vi "CRC.vi"(9 "length":i32=496, 10 "index":i32=20, 11 "DS5CalibrationCoefficientsTable":u8[](array[numeric])=[21, 0, 0, 0, 3, 0, 25, 0, 240, 1, 0, 0, 0, 4, 0, 4, 169, 238, 63, 236, 156, 141, 55, 63, 113, 190, 162, 63, 135, 142, 252, 62, 9, 233, 5, 63, 31, 150, 10, 62, 55, 118, 207, 190, 113, 68, 102, 58, 249, 138, 146, 186, 37, 191, 183, 62, 140, 183, 56, 63, 9, 210, 163, 63, 166, 65, 2, 63, 224, 139, 1, 63, 100, 118, 2, 62, 234, 150, 203, 190, 17, 251, 198, 57, 162, 214, 21, 187, 174, 168, 180, 62, 233, 255, 127, 63, 123, 123, 122, 58, 169, 40, 178, 186, 91, 254, 122, 186, 231, 255, 127, 63, 249, 16, 188, 186, 151, 250, 177, 58, 148, 60, 188, 58, 223, 255, 127, 63, 253, 254, 127, 63, 187, 169, 2, 187, 133, 7, 170, 187, 170, 38, 3, 59, 205, 255, 127, 63, 195, 120, 187, 58, 120, 239, 169, 59, 115, 212, 188, 186, 13, 255, 127, 63, 197, 83, 91, 194, 1, 0, 0, 0, 0, 0, 0, 0, 0, 0, 0, 0, 0, 0, 0, 0, 0, 0, 0, 0, 0, 0, 0, 0, 0, 0, 0, 0, 0, 0, 0, 0, 0, 0, 0, 0, 0, 0, 0, 0, 0, 0, 0, 0, 0, 0, 0, 0, 0, 0, 0, 0, 0, 0, 0, 0, 0, 0, 0, 0, 0, 0, 0, 0, 0, 0, 0, 0, 0, 0, 0, 0, 0, 0, 0, 0, 0, 0, 0, 0, 0, 0, 0, 0, 0, 0, 0, 0, 0, 0, 0, 0, 27, 157, 178, 68, 27, 157, 178, 68, 254, 246, 109, 68, 45, 3, 11, 68, 207, 38, 110, 68, 207, 38, 110, 68, 169, 164, 30, 68, 145, 89, 185, 67, 138, 196, 30, 68, 138, 196, 30, 68, 225, 48, 158, 67, 23, 34, 119, 67, 138, 196, 30, 68, 138, 196, 30, 68, 225, 48, 210, 67, 23, 34, 119, 67, 207, 38, 238, 67, 207, 38, 238, 67, 169, 164, 158, 67, 145, 89, 57, 67, 138, 196, 158, 67, 138, 196, 158, 67, 225, 48, 82, 67, 23, 34, 247, 66, 138, 196, 158, 67, 138, 196, 158, 67, 225, 48, 30, 67, 23, 34, 247, 66, 27, 157, 178, 67, 27, 157, 178, 67, 254, 246, 109, 67, 45, 3, 11, 67, 115, 78, 132, 68, 115, 78, 132, 68, 17, 126, 30, 68, 190, 241, 205, 67, 27, 157, 50, 68, 27, 157, 50, 68, 254, 246, 237, 67, 45, 3, 139, 67, 0, 0, 0, 0, 0, 0, 0, 0, 0, 0, 0, 0, 0, 0, 0, 0, 0, 0, 0, 0, 0, 0, 0, 0, 0, 0, 0, 0, 0, 0, 0, 0, 0, 0, 0, 0, 0, 0, 0, 0, 0, 0, 0, 0, 0, 0, 0, 0, 0, 0, 0, 0, 0, 0, 0, 0, 0, 0, 0, 0, 0, 0, 0, 0, 0, 0, 0, 0, 0, 0, 0, 0, 0, 0, 0, 0, 0, 0, 0, 0, 0, 0, 0, 0, 0, 0, 0, 0, 0, 0, 0, 0, 0, 0, 0, 0, 0, 0, 0, 0, 105, 207, 27, 52, 0, 14, 0, 128, 67, 0, 58, 0, 92, 0, 80, 0, 114, 0, 111, 0, 103, 0, 114, 0, 97, 0, 109, 0, 32, 0, 70, 0, 105, 0, 108, 0, 101, 0, 115, 0, 92, 0, 78, 0, 97, 0, 116, 0, 105, 0, 111, 0, 110, 0, 97, 0, 108, 0, 32, 0, 73, 0, 110, 0, 115, 0, 116, 0, 114, 0, 117, 0, 109, 0, 101, 0, 110, 0, 116, 0, 115, 0, 92, 0, 76, 0, 97, 0, 98, 0, 86, 0, 73, 0, 69, 0, 87, 0, 32, 0, 50, 0, 48, 0, 49, 0, 54, 0, 92, 0, 76, 0, 97, 0, 98, 0, 86, 0, 73, 0, 69, 0, 87, 0, 46, 0, 101, 0, 120, 0, 101, 0, 0, 0, 114, 0, 101, 0, 92, 0, 112, 0, 110, 0, 103, 0, 46, 0, 108, 0, 108, 0, 98, 0, 0, 0, 0, 0, 0, 0, 0, 0, 0, 0, 0, 0, 0, 0, 0, 0, 0, 0, 0, 0, 0, 0, 0, 0, 0, 0, 0, 0, 0, 0, 0, 0, 0, 0, 0, 0, 0, 0, 0, 0, 0, 0, 0, 0, 0, 0, 0, 0, 0, 0, 0, 0, 0, 0, 0, 0, 0, 0, 0, 0, 0, 0, 0, 0, 0, 0, 0, 0, 0, 0, 0, 0, 0, 0, 0, 0, 0, 0, 0, 0, 0, 0, 0, 0, 0, 0, 0, 0, 0, 0, 0, 0, 0, 0, 0, 0, 0, 0, 0, 0, 0, 0, 0, 0, 0, 0, 0, 0, 0, 0, 0, 0, 0, 0, 0, 0, 0, 0, 0, 0, 0, 0, 0, 0, 0, 0, 0, 0, 0, 0, 0, 0, 0, 0, 0, 0, 0, 0, 0, 0, 0, 0, 0, 0, 0, 0, 0, 0, 0, 0, 0, 0, 0, 0, 0, 0, 0, 0, 0, 0, 0, 0, 0, 0, 0, 0, 0, 0, 0, 0, 0, 0, 0, 0, 0, 0, 0, 0, 0, 0, 0, 0, 0, 0, 0, 0, 0, 0, 0, 0, 0, 0, 0, 0, 0, 0, 0, 0, 0, 0, 0, 0, 0, 0, 0, 0, 0, 0, 0, 0, 0, 0, 0, 0, 0, 0, 0, 0, 0, 0, 0, 0, 0, 0, 0, 0, 0, 0, 0, 0, 0, 0, 0, 0, 0, 0, 0, 0, 0, 0, 0, 0, 0, 0, 0, 0, 0, 0, 0, 0, 0, 0, 0, 0, 0, 0, 0, 0, 0, 0, 0, 0, 0, 0, 0, 0, 0, 0, 0, 0, 0, 0, 0, 0, 0, 0, 0, 0, 0, 0, 0, 0, 0, 0, 0, 0, 0, 0, 0, 0, 0, 0, 0, 0, 0, 0, 0, 0, 0, 0, 0, 0, 0, 0, 0, 0, 0, 0, 0, 0, 0, 0, 0, 0, 0, 0, 0, 0, 0, 0, 0, 0, 0, 0, 0, 0, 0, 0, 0, 0, 0, 0, 0, 0, 0, 0, 0, 0, 0, 0, 0, 0, 0, 0, 0, 0, 0, 0, 0, 0] format="%x") -> (2 "CRC array":u8[](array[numeric]), 3 "CRC output":u32=3963612841 format="%x")   [LabVIEW 2017, in "libRealSense3.lvlib"]
uses:
  libRealSense3.lvlib
panel:
  out "Calibration table":T1={"version"=3, "table type"=60479, "table size"=496, "full version"=67109888, "crc32"=3963612841, "baseline"=-54.831806, "model"=1, "fx left"=917.7658, "fy left"=915.4345, "px left"=631.39185, "py left"=376.6227, "py right"=364.3492, "px right"=651.2822, "fy right"=921.49005, "fx right"=923.5849, "k left"=[0.13533829, -0.40519878, 0.0008784002, -0.0011180333, 0.3588802], "k right"=[0.12740475, -0.39763576, 0.00037952562, -0.0022863527, 0.35284942], "RLeft"=[0.9999986, 0.0009555143, -0.001359244, -0.0009574645, 0.9999985, -0.001434832, 0.001357871, 0.0014361315, 0.99999803], "Rright"=[0.99998456, -0.0019937593, -0.0051888847, 0.002001206, 0.99999696, 0.0014302958, 0.0051860176, -0.0014406577, 0.9999855], "uint8 reserved1"=[0, 0, 0, 0, 0, 0, 0, 0, 0, 0, 0, 0, 0, 0, 0, 0, 0, 0, 0, 0, 0, 0, 0, 0, 0, 0, 0, 0, 0, 0, 0, 0, 0, 0, 0, 0, 0, 0, 0, 0, 0, 0, 0, 0, 0, 0, 0, 0, 0, 0, 0, 0, 0, 0, 0, 0, 0, 0, 0, 0, 0, 0, 0, 0, 0, 0, 0, 0, 0, 0, 0, 0, 0, 0, 0, 0, 0, 0, 0, 0, 0, 0, 0, 0, 0, 0, 0, 0], "uint8 reserved2"=[0, 0, 0, 0, 0, 0, 0, 0, 0, 0, 0, 0, 0, 0, 0, 0, 0, 0, 0, 0, 0, 0, 0, 0, 0, 0, 0, 0, 0, 0, 0, 0, 0, 0, 0, 0, 0, 0, 0, 0, 0, 0, 0, 0, 0, 0, 0, 0, 0, 0, 0, 0, 0, 0, 0, 0, 0, 0, 0, 0, 0, 0, 0, 0], "1920x1080"=[1428.9095, 1428.9095, 951.85925, 556.0496], "1280x720"=[952.6064, 952.6064, 634.5728, 370.69974], "640x480"=[635.0709, 635.0709, 316.38187, 247.13316], "848x480"=[635.0709, 635.0709, 420.38187, 247.13316], "640x360"=[476.3032, 476.3032, 317.2864, 185.34987], "424x240"=[317.53546, 317.53546, 210.19093, 123.56658], "320x240"=[317.53546, 317.53546, 158.19093, 123.56658], "480x270"=[357.2274, 357.2274, 237.96481, 139.0124], "1280x800"=[1058.4515, 1058.4515, 633.9698, 411.8886], "960x540"=[714.4548, 714.4548, 475.92963, 278.0248], "Reserved1"=[714.4548, 714.4548, 475.92963, 278.0248], "Reserved 2"=[714.4548, 714.4548, 475.92963, 278.0248]} {"crc32" format="%x"}
  out "iteration":i32=495
  out "CRC Array":u32[](array[numeric])=[0, 1996959894, 3993919788, 2567524794, 124634137, 1886057615, 3915621685, 2657392035, 249268274, 2044508324, 3772115230, 2547177864, 162941995, 2125561021, 3887607047, 2428444049, 498536548, 1789927666, 4089016648, 2227061214, 450548861, 1843258603, 4107580753, 2211677639, 325883990, 1684777152, 4251122042, 2321926636, 335633487, 1661365465, 4195302755, 2366115317, 997073096, 1281953886, 3579855332, 2724688242, 1006888145, 1258607687, 3524101629, 2768942443, 901097722, 1119000684, 3686517206, 2898065728, 853044451, 1172266101, 3705015759, 2882616665, 651767980, 1373503546, 3369554304, 3218104598, 565507253, 1454621731, 3485111705, 3099436303, 671266974, 1594198024, 3322730930, 2970347812, 795835527, 1483230225, 3244367275, 3060149565, 1994146192, 31158534, 2563907772, 4023717930, 1907459465, 112637215, 2680153253, 3904427059, 2013776290, 251722036, 2517215374, 3775830040, 2137656763, 141376813, 2439277719, 3865271297, 1802195444, 476864866, 2238001368, 4066508878, 1812370925, 453092731, 2181625025, 4111451223, 1706088902, 314042704, 2344532202, 4240017532, 1658658271, 366619977, 2362670323, 4224994405, 1303535960, 984961486, 2747007092, 3569037538, 1256170817, 1037604311, 2765210733, 3554079995, 1131014506, 879679996, 2909243462, 3663771856, 1141124467, 855842277, 2852801631, 3708648649, 1342533948, 654459306, 3188396048, 3373015174, 1466479909, 544179635, 3110523913, 3462522015, 1591671054, 702138776, 2966460450, 3352799412, 1504918807, 783551873, 3082640443, 3233442989, 3988292384, 2596254646, 62317068, 1957810842, 3939845945, 2647816111, 81470997, 1943803523, 3814918930, 2489596804, 225274430, 2053790376, 3826175755, 2466906013, 167816743, 2097651377, 4027552580, 2265490386, 503444072, 1762050814, 4150417245, 2154129355, 426522225, 1852507879, 4275313526, 2312317920, 282753626, 1742555852, 4189708143, 2394877945, 397917763, 1622183637, 3604390888, 2714866558, 953729732, 1340076626, 3518719985, 2797360999, 1068828381, 1219638859, 3624741850, 2936675148, 906185462, 1090812512, 3747672003, 2825379669, 829329135, 1181335161, 3412177804, 3160834842, 628085408, 1382605366, 3423369109, 3138078467, 570562233, 1426400815, 3317316542, 2998733608, 733239954, 1555261956, 3268935591, 3050360625, 752459403, 1541320221, 2607071920, 3965973030, 1969922972, 40735498, 2617837225, 3943577151, 1913087877, 83908371, 2512341634, 3803740692, 2075208622, 213261112, 2463272603, 3855990285, 2094854071, 198958881, 2262029012, 4057260610, 1759359992, 534414190, 2176718541, 4139329115, 1873836001, 414664567, 2282248934, 4279200368, 1711684554, 285281116, 2405801727, 4167216745, 1634467795, 376229701, 2685067896, 3608007406, 1308918612, 956543938, 2808555105, 3495958263, 1231636301, 1047427035, 2932959818, 3654703836, 1088359270, 936918000, 2847714899, 3736837829, 1202900863, 817233897, 3183342108, 3401237130, 1404277552, 615818150, 3134207493, 3453421203, 1423857449, 601450431, 3009837614, 3294710456, 1567103746, 711928724, 3020668471, 3272380065, 1510334235, 755167117] format="%x"
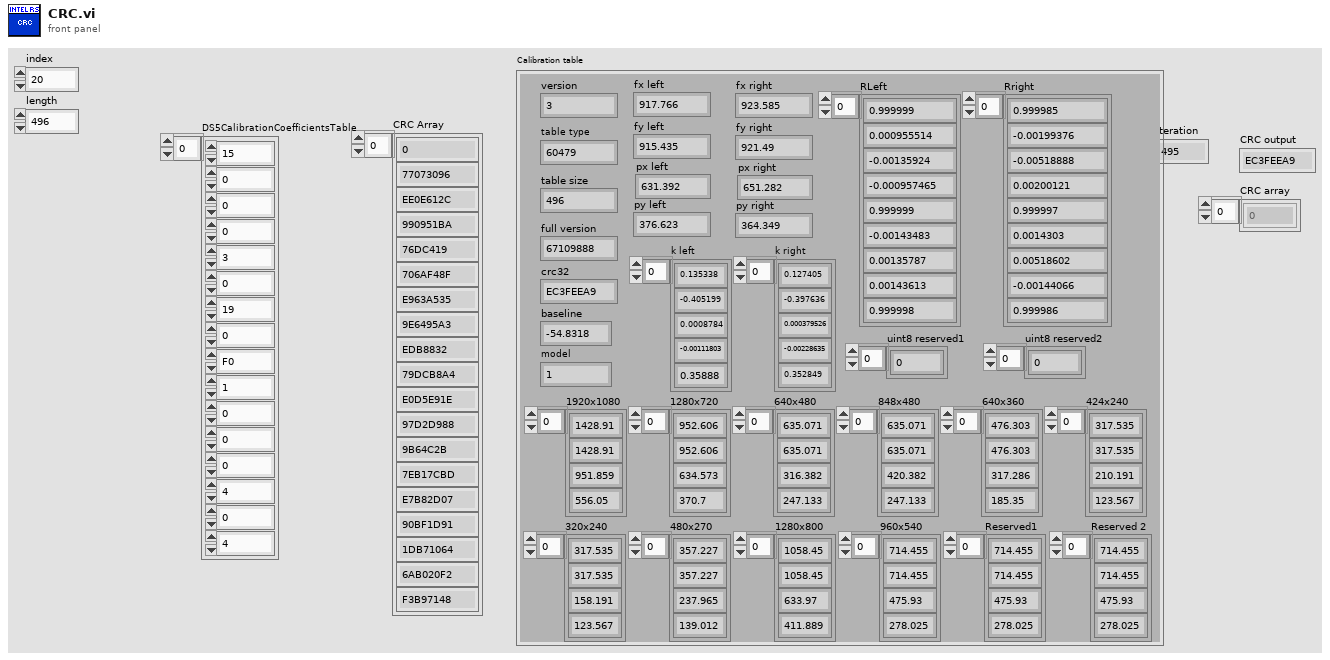
[diagram p1: front panel]
types:
  T1 = cluster{"version":u16, "table type":u16, "table size":u32, "full version":u32, "crc32":u32, "baseline":sgl, "model":u32, "fx left":sgl, "fy left":sgl, "px left":sgl, "py left":sgl, "py right":sgl, "px right":sgl, "fy right":sgl, "fx right":sgl, "k left":sgl[], "k right":sgl[], "RLeft":sgl[], "Rright":sgl[], "uint8 reserved1":u8[], "uint8 reserved2":u8[], "1920x1080":sgl[], "1280x720":sgl[], "640x480":sgl[], "848x480":sgl[], "640x360":sgl[], "424x240":sgl[], "320x240":sgl[], "480x270":sgl[], "1280x800":sgl[], "960x540":sgl[], "Reserved1":sgl[], "Reserved 2":sgl[]}
  T2 = enum16{"big-endian, network order", "native, host order", "little-endian"}
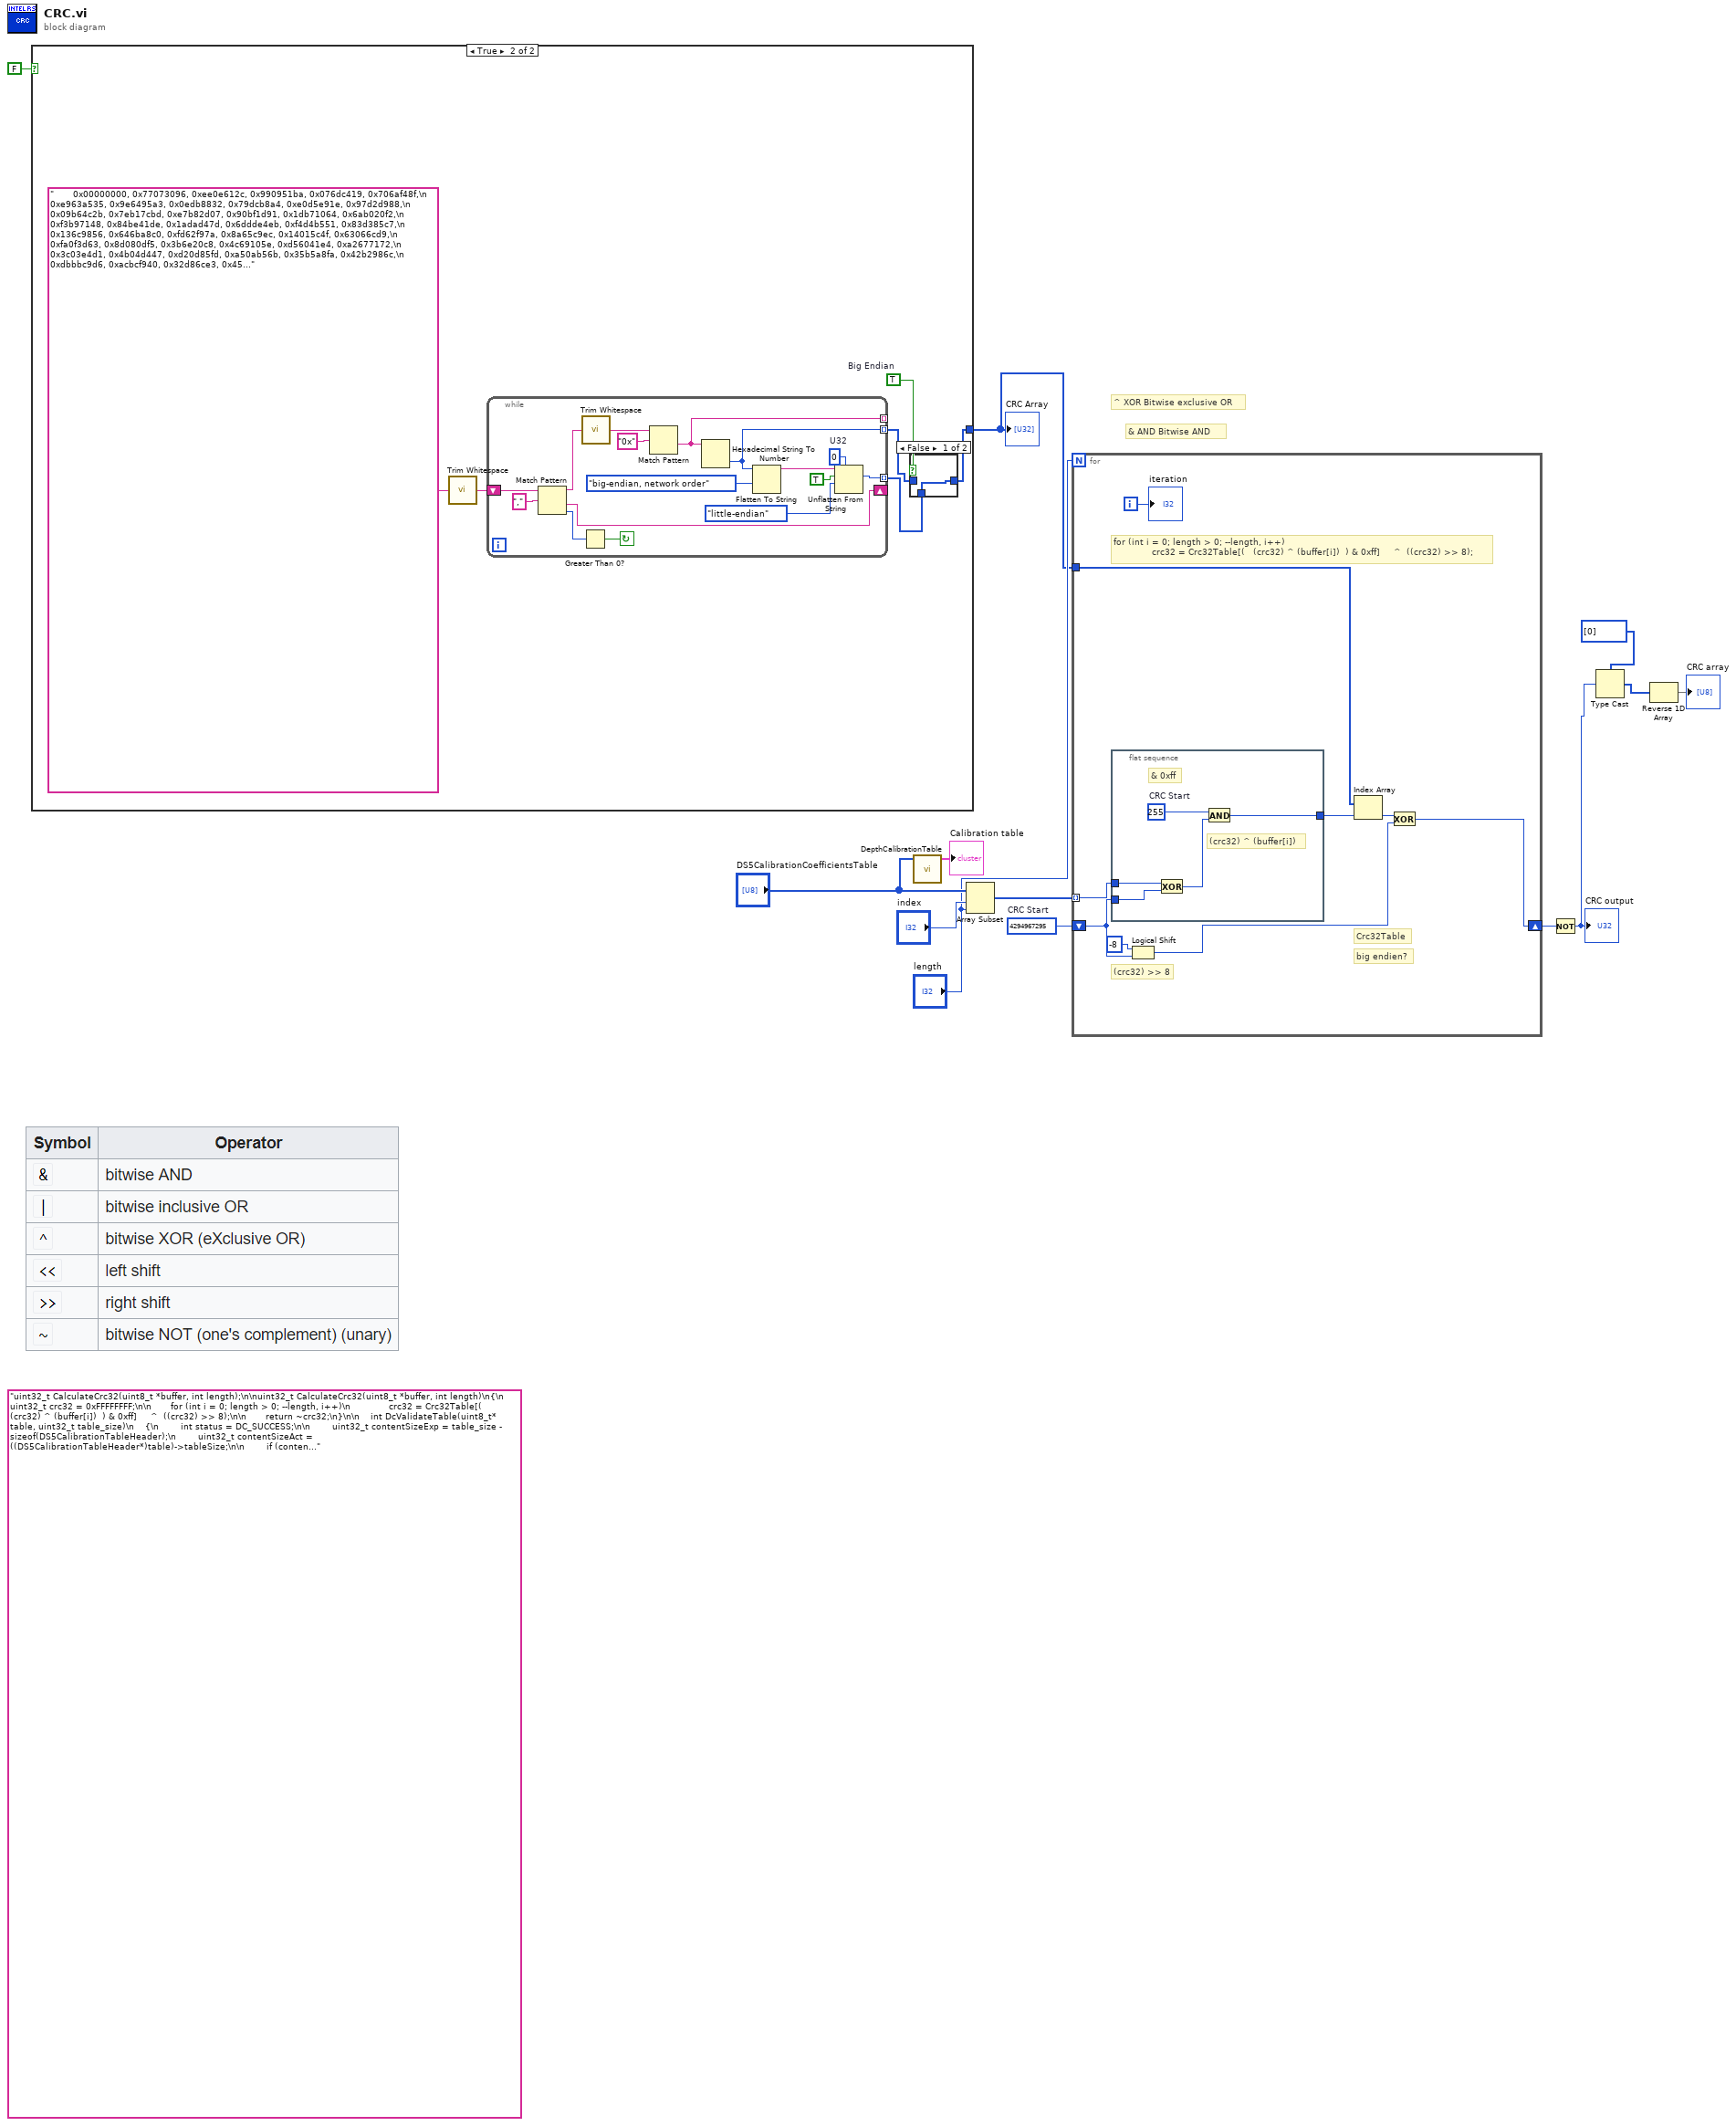
[diagram p0: block diagram]
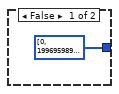
[diagram p2: hidden frame]
diagram:
  w13 = u32 4294967295  # CRC Start
  (unwired) "uint32_t CalculateCrc32(uint8_t *buffer, int length);\n\nuint32_t CalculateCrc32(uint8_t *buffer, int length)\n{\n       uint32_t crc32 = 0xFFFFFFFF;\n\n       for (int i = 0; length > 0; --length, i++)\n              crc32 = Crc32Table[(   (crc32) ^ (buffer[i])  ) & 0xff]     ^  ((crc32) >> 8);\n\n       return ~crc32;\n}\n\n    int DcValidateTable(uint8_t* table, uint32_t table_size)\n    {\n        int status = DC_SUCCESS;\n\n        uint32_t contentSizeExp = table_size - sizeof(DS5CalibrationTableHeader);\n        uint32_t contentSizeAct = ((DS5CalibrationTableHeader*)table)->tableSize;\n\n        if (contentSizeAct > contentSizeExp )\n        {\n            return DC_ERROR_MISMATCH_CAL_TABLE_SIZE;\n        }\n\n        uint8_t* content = table + sizeof(DS5CalibrationTableHeader);\n        uint32_t crc32_comp = CalculateCrc32(content, contentSizeAct);\n        uint32_t crc32_act  = ((DS5CalibrationTableHeader *)table)->crc32;\n\n        if (crc32_act != crc32_comp)\n       {\n            status = DC_ERROR_MISMATCH_CAL_TABLE_CRC;\n        }\n\n        return status;\n       }\n\n\nstruct MMTableHeader\n{\n       uint16_t version;                       //!< Table version\n       uint16_t tableType;                     //!< Table type\n       uint32_t tableSize;                     //!< Table size\n       uint32_t resrved;                       //!< reserved field\n       uint32_t crc32;                         //!< CRC32 of the content\n};\n\n\n\n\n\n\n            status = DcValidateTable(buffer, sizeof(DS5CoefficientsParamsTable));\n"
  # "&\tAND\tBitwise AND"
  # "^\tXOR\tBitwise exclusive OR"
  n1 = case shown="True" FALSE {
    tunnel: [u32[] [0, 1996959894, 3993919788, 2567524794, 124634137, 1886057615, 3915621685, 2657392035, 249268274, 2044508324, 3772115230, 2547177864, 162941995, 2125561021, 3887607047, 2428444049, 498536548, 1789927666, 4089016648, 2227061214, 450548861, 1843258603, 4107580753, 2211677639, 325883990, 1684777152, 4251122042, 2321926636, 335633487, 1661365465, 4195302755, 2366115317, 997073096, 1281953886, 3579855332, 2724688242, 1006888145, 1258607687, 3524101629, 2768942443, 901097722, 1119000684, 3686517206, 2898065728, 853044451, 1172266101, 3705015759, 2882616665, 651767980, 1373503546, 3369554304, 3218104598, 565507253, 1454621731, 3485111705, 3099436303, 671266974, 1594198024, 3322730930, 2970347812, 795835527, 1483230225, 3244367275, 3060149565, 1994146192, 31158534, 2563907772, 4023717930, 1907459465, 112637215, 2680153253, 3904427059, 2013776290, 251722036, 2517215374, 3775830040, 2137656763, 141376813, 2439277719, 3865271297, 1802195444, 476864866, 2238001368, 4066508878, 1812370925, 453092731, 2181625025, 4111451223, 1706088902, 314042704, 2344532202, 4240017532, 1658658271, 366619977, 2362670323, 4224994405, 1303535960, 984961486, 2747007092, 3569037538, 1256170817, 1037604311, 2765210733, 3554079995, 1131014506, 879679996, 2909243462, 3663771856, 1141124467, 855842277, 2852801631, 3708648649, 1342533948, 654459306, 3188396048, 3373015174, 1466479909, 544179635, 3110523913, 3462522015, 1591671054, 702138776, 2966460450, 3352799412, 1504918807, 783551873, 3082640443, 3233442989, 3988292384, 2596254646, 62317068, 1957810842, 3939845945, 2647816111, 81470997, 1943803523, 3814918930, 2489596804, 225274430, 2053790376, 3826175755, 2466906013, 167816743, 2097651377, 4027552580, 2265490386, 503444072, 1762050814, 4150417245, 2154129355, 426522225, 1852507879, 4275313526, 2312317920, 282753626, 1742555852, 4189708143, 2394877945, 397917763, 1622183637, 3604390888, 2714866558, 953729732, 1340076626, 3518719985, 2797360999, 1068828381, 1219638859, 3624741850, 2936675148, 906185462, 1090812512, 3747672003, 2825379669, 829329135, 1181335161, 3412177804, 3160834842, 628085408, 1382605366, 3423369109, 3138078467, 570562233, 1426400815, 3317316542, 2998733608, 733239954, 1555261956, 3268935591, 3050360625, 752459403, 1541320221, 2607071920, 3965973030, 1969922972, 40735498, 2617837225, 3943577151, 1913087877, 83908371, 2512341634, 3803740692, 2075208622, 213261112, 2463272603, 3855990285, 2094854071, 198958881, 2262029012, 4057260610, 1759359992, 534414190, 2176718541, 4139329115, 1873836001, 414664567, 2282248934, 4279200368, 1711684554, 285281116, 2405801727, 4167216745, 1634467795, 376229701, 2685067896, 3608007406, 1308918612, 956543938, 2808555105, 3495958263, 1231636301, 1047427035, 2932959818, 3654703836, 1088359270, 936918000, 2847714899, 3736837829, 1202900863, 817233897, 3183342108, 3401237130, 1404277552, 615818150, 3134207493, 3453421203, 1423857449, 601450431, 3009837614, 3294710456, 1567103746, 711928724, 3020668471, 3272380065, 1510334235, 755167117] ("CRC Array") w16] -> w6
    frame False {
    }
    frame True {
      w18 = TRUE  # Big Endian
      n2 = call <vilib>:"Trim Whitespace.vi"("string"="       0x00000000, 0x77073096, 0xee0e612c, 0x990951ba, 0x076dc419, 0x706af48f,\n       0xe963a535, 0x9e6495a3, 0x0edb8832, 0x79dcb8a4, 0xe0d5e91e, 0x97d2d988,\n       0x09b64c2b, 0x7eb17cbd, 0xe7b82d07, 0x90bf1d91, 0x1db71064, 0x6ab020f2,\n       0xf3b97148, 0x84be41de, 0x1adad47d, 0x6ddde4eb, 0xf4d4b551, 0x83d385c7,\n       0x136c9856, 0x646ba8c0, 0xfd62f97a, 0x8a65c9ec, 0x14015c4f, 0x63066cd9,\n       0xfa0f3d63, 0x8d080df5, 0x3b6e20c8, 0x4c69105e, 0xd56041e4, 0xa2677172,\n       0x3c03e4d1, 0x4b04d447, 0xd20d85fd, 0xa50ab56b, 0x35b5a8fa, 0x42b2986c,\n       0xdbbbc9d6, 0xacbcf940, 0x32d86ce3, 0x45df5c75, 0xdcd60dcf, 0xabd13d59,\n       0x26d930ac, 0x51de003a, 0xc8d75180, 0xbfd06116, 0x21b4f4b5, 0x56b3c423,\n       0xcfba9599, 0xb8bda50f, 0x2802b89e, 0x5f058808, 0xc60cd9b2, 0xb10be924,\n       0x2f6f7c87, 0x58684c11, 0xc1611dab, 0xb6662d3d, 0x76dc4190, 0x01db7106,\n       0x98d220bc, 0xefd5102a, 0x71b18589, 0x06b6b51f, 0x9fbfe4a5, 0xe8b8d433,\n       0x7807c9a2, 0x0f00f934, 0x9609a88e, 0xe10e9818, 0x7f6a0dbb, 0x086d3d2d,\n       0x91646c97, 0xe6635c01, 0x6b6b51f4, 0x1c6c6162, 0x856530d8, 0xf262004e,\n       0x6c0695ed, 0x1b01a57b, 0x8208f4c1, 0xf50fc457, 0x65b0d9c6, 0x12b7e950,\n       0x8bbeb8ea, 0xfcb9887c, 0x62dd1ddf, 0x15da2d49, 0x8cd37cf3, 0xfbd44c65,\n       0x4db26158, 0x3ab551ce, 0xa3bc0074, 0xd4bb30e2, 0x4adfa541, 0x3dd895d7,\n       0xa4d1c46d, 0xd3d6f4fb, 0x4369e96a, 0x346ed9fc, 0xad678846, 0xda60b8d0,\n       0x44042d73, 0x33031de5, 0xaa0a4c5f, 0xdd0d7cc9, 0x5005713c, 0x270241aa,\n       0xbe0b1010, 0xc90c2086, 0x5768b525, 0x206f85b3, 0xb966d409, 0xce61e49f,\n       0x5edef90e, 0x29d9c998, 0xb0d09822, 0xc7d7a8b4, 0x59b33d17, 0x2eb40d81,\n       0xb7bd5c3b, 0xc0ba6cad, 0xedb88320, 0x9abfb3b6, 0x03b6e20c, 0x74b1d29a,\n       0xead54739, 0x9dd277af, 0x04db2615, 0x73dc1683, 0xe3630b12, 0x94643b84,\n       0x0d6d6a3e, 0x7a6a5aa8, 0xe40ecf0b, 0x9309ff9d, 0x0a00ae27, 0x7d079eb1,\n       0xf00f9344, 0x8708a3d2, 0x1e01f268, 0x6906c2fe, 0xf762575d, 0x806567cb,\n       0x196c3671, 0x6e6b06e7, 0xfed41b76, 0x89d32be0, 0x10da7a5a, 0x67dd4acc,\n       0xf9b9df6f, 0x8ebeeff9, 0x17b7be43, 0x60b08ed5, 0xd6d6a3e8, 0xa1d1937e,\n       0x38d8c2c4, 0x4fdff252, 0xd1bb67f1, 0xa6bc5767, 0x3fb506dd, 0x48b2364b,\n       0xd80d2bda, 0xaf0a1b4c, 0x36034af6, 0x41047a60, 0xdf60efc3, 0xa867df55,\n       0x316e8eef, 0x4669be79, 0xcb61b38c, 0xbc66831a, 0x256fd2a0, 0x5268e236,\n       0xcc0c7795, 0xbb0b4703, 0x220216b9, 0x5505262f, 0xc5ba3bbe, 0xb2bd0b28,\n       0x2bb45a92, 0x5cb36a04, 0xc2d7ffa7, 0xb5d0cf31, 0x2cd99e8b, 0x5bdeae1d,\n       0x9b64c2b0, 0xec63f226, 0x756aa39c, 0x026d930a, 0x9c0906a9, 0xeb0e363f,\n       0x72076785, 0x05005713, 0x95bf4a82, 0xe2b87a14, 0x7bb12bae, 0x0cb61b38,\n       0x92d28e9b, 0xe5d5be0d, 0x7cdcefb7, 0x0bdbdf21, 0x86d3d2d4, 0xf1d4e242,\n       0x68ddb3f8, 0x1fda836e, 0x81be16cd, 0xf6b9265b, 0x6fb077e1, 0x18b74777,\n       0x88085ae6, 0xff0f6a70, 0x66063bca, 0x11010b5c, 0x8f659eff, 0xf862ae69,\n       0x616bffd3, 0x166ccf45, 0xa00ae278, 0xd70dd2ee, 0x4e048354, 0x3903b3c2,\n       0xa7672661, 0xd06016f7, 0x4969474d, 0x3e6e77db, 0xaed16a4a, 0xd9d65adc,\n       0x40df0b66, 0x37d83bf0, 0xa9bcae53, 0xdebb9ec5, 0x47b2cf7f, 0x30b5ffe9,\n       0xbdbdf21c, 0xcabac28a, 0x53b39330, 0x24b4a3a6, 0xbad03605, 0xcdd70693,\n       0x54de5729, 0x23d967bf, 0xb3667a2e, 0xc4614ab8, 0x5d681b02, 0x2a6f2b94,\n       0xb40bbe37, 0xc30c8ea1, 0x5a05df1b, 0x2d02ef8d\n") -> ("trimmed string"=w19:string)  [unwired: 1 in]
      n3 = while {
        shift-right: [w34] -> _
        shift-left: w19 -> [w38]
        tunnel: [w25] -> w17 mode=indexing
        tunnel: [w27] -> w15 mode=indexing
        tunnel: [w26] -> _ mode=indexing
        stop <- w35 continue-if-true
        w28 = u32 0  # U32
        n4 = Match Pattern(string=w38, regular expression=",") -> (before substring=w33:string, after substring=w34:string, offset past match=w36:i32)  [unwired: 1 in, 1 out]
        n5 = Greater Than 0?(x=w36) -> (x > 0?=w35:bool)
        n6 = call <vilib>:"Trim Whitespace.vi"("string"=w33) -> ("trimmed string"=w32:string)  [unwired: 1 in]
        n7 = Match Pattern(string=w32, regular expression="0x" ("substring (\"\")")) -> (after substring=w26:string)  [unwired: 1 in, 3 out]
        n8 = Hexadecimal String To Number(string=w26) -> (number=w25:u32)  [unwired: 2 in, 1 out]
        n9 = Flatten To String(anything=w25, byte order (0:big-endian, network order)=T2."big-endian, network order") -> (data string=w23:string)  [unwired: 2 in, 2 out]
        n10 = Unflatten From String(type=w28, binary string=w23, data includes array or string size? (T)=TRUE, byte order (0:big-endian, network order)=T2."little-endian") -> (value=w27:u32)  [unwired: 1 in, 2 out]
      }
      n11 = case shown="False" w18 {
        tunnel: w17 -> [_ w22]
        tunnel: [w21 w22] -> w16
        tunnel: w15 -> [w21 _]
        frame False {
        }
        frame True {
        }
      }
    }
  }
  "CRC Array" <- w6
  n12 = call "DepthCalibrationTable.vi"("DS5CalibrationCoefficientsTable"="DS5CalibrationCoefficientsTable") -> ("Calibration table"=→"Calibration table":T1)  [unwired: 7 in, 3 out]
  n13 = Array Subset(array="DS5CalibrationCoefficientsTable", index="index", length="length") -> (w10:u8[])
  n14 = for {
    N: "length" -> [_]
    tunnel: w10 -> [w47] mode=indexing
    shift-right: [w40] -> w12
    shift-left: w13 -> [w44]
    tunnel: w6 -> [w46]
    i -> [w39]
    # "big endien?"
    # "Crc32Table"
    # "(crc32) >> 8"
    # "for (int i = 0; length > 0; --length, i++)\n              crc32 = Crc32Table[(   (crc32) ^ (buffer[i])  ) & 0xff]     ^  ((crc32) >> 8);"
    n15 = flat-sequence {
      tunnel: w47 -> [w52]
      tunnel: [w49] -> w45
      tunnel: w44 -> [w48]
      frame #0 {
        w50 = u32 255  # CRC Start
        # "& 0xff"
        # "(crc32) ^ (buffer[i])"
        n16 = Exclusive Or(1:w48, 2:w52) -> (0:w51:u32)
        n17 = And(x=w50, y=w51) -> (x .and. y?=w49:u32)
      }
    }
    n18 = Logical Shift(y=-8 ("x"), x=w44) -> (x << y=w42:u32)
    n19 = Index Array(array=w46, index=w45) -> (element=w41:u32)
    n20 = Exclusive Or(1:w42, 2:w41) -> (0:w40:u32)
    "iteration" <- w39
  }
  n21 = Not(x=w12) -> (.not. x?=w4:u32)
  "CRC output" <- w4
  n22 = Type Cast(type=u8[] [0], x=w4) -> (*(type *) &x=w3:u8[])
  n23 = Reverse 1D Array(array=w3) -> (reversed array=→"CRC array":u8[])
